vi "uTransport_IsValid.vi"(8 "error in (no error)":errorcluster, 11 "uTransport_Event in":refnum<class "uTransport_Event.lvclass">) -> (0 "error out":errorcluster, 2 "IsValid?":bool, 3 "uTransport_Event out":refnum<class "uTransport_Event.lvclass">)   [LabVIEW 2021, in "uFramework.lvlib" / "uTransport_Event.lvclass"]
uses:
  uTransport_Event.lvclass
  uTransport_Event.lvclass/uTransport_Event.ctl
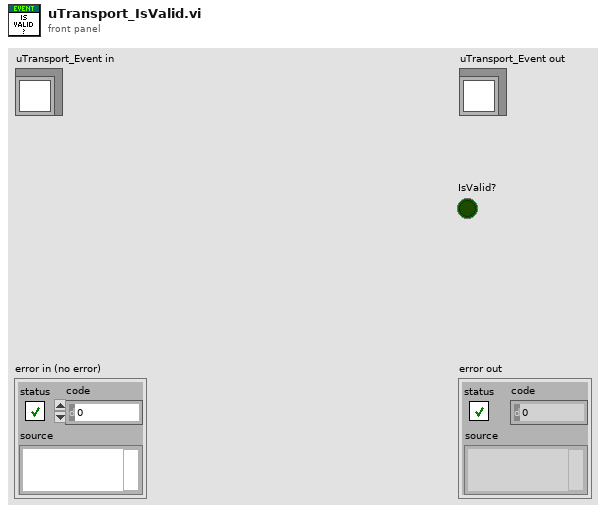
[diagram p1: front panel]
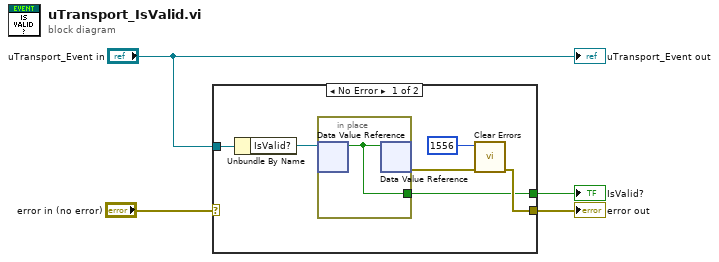
[diagram p0: block diagram]
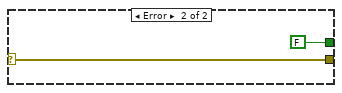
[diagram p2: hidden frame]
diagram:
  n1 = case shown="No Error" "error in (no error)" {
    selector: "error in (no error)" -> [_ w12]
    tunnel: "uTransport_Event in" -> [w5 _]
    tunnel: [w7 FALSE ("Is Valid?")] -> w3
    tunnel: [w10 w12] -> w2
    frame No Error {
      n2 = Unbundle By Name(w5) -> ("IsValid?"=w8:refnum<data-value>)
      n3 = in-place {
        in-place-border: [w11] -> w7
        n4 = in-place-dvr #1(w8) -> (w11:bool)  [unwired: 1 out]
        n5 = in-place-dvr #1(w11) -> (w6:errorcluster)  [unwired: 1 out]
      }
      n6 = call <vilib>:"Clear Errors.vi"("error in (no error)"=w6, "specific error code to clear (0: all)"=1556) -> ("error out"=w10:errorcluster)  [unwired: 4 in, 1 out]
    }
    frame Error {
    }
  }
  "error out" <- w2
  "IsValid?" <- w3
  "uTransport_Event out" <- "uTransport_Event in"
